vi "SenseQuiet_correct_final one.vi"() -> ()   [LabVIEW 2020]
uses:
  <vilib>/Platform/TimedLoop/XDataNode/timing_clust.ctl
  <vilib>/Platform/TimedLoop/XDataNode/nitl_modes.ctl
  <vilib>/Platform/TimedLoop/XDataNode/wakeup.ctl
  <vilib>/Instr/_visa.llb/VISA Configure Serial Port (Instr).vi
  <vilib>/platform/TimedLoop/XDataNode/XDataNode.xnode
  <vilib>/Platform/TimedLoop/XDataNode/XDNodeRunTimeDep.lvlib
  <vilib>/ptbypt/NI_PtbyPt.lvlib
panel:
  in  "OLED Display Output":refnum<visa-resource-name>
  out "WARNING":string="Warning - Please be mindful of noise"
  out "VIOLATION":string="Violation! - Noise Level too high"
  out "WARNING":string="Warning - A Noise Persisting"
  out "CALIBRATING":string="Calibrating"
  out "Sound Waveform":dynamicdata(graph) caption="Sound Sensor Output"
  out "PIR Sensor":bool
  out "Light Sensor":bool
  in  "Case Structure Loop Stop":bool
  in  "Main Loop Stop":bool
  out "Violation Noise Elapsed Time":dbl caption="Elapsed Time (s)"
  out "Violation Threshold":dbl
  out "Warning Threshold":dbl
  out "Noise Floor":dbl
  out "Noise Level Over Time":dbl(graph)
  out "System Message":string
  out "Buzzer Active":bool
  out "Violation LED":bool
  out "Warning LED":bool
  out "Quiet LED":bool
  # "SenseQuiet"
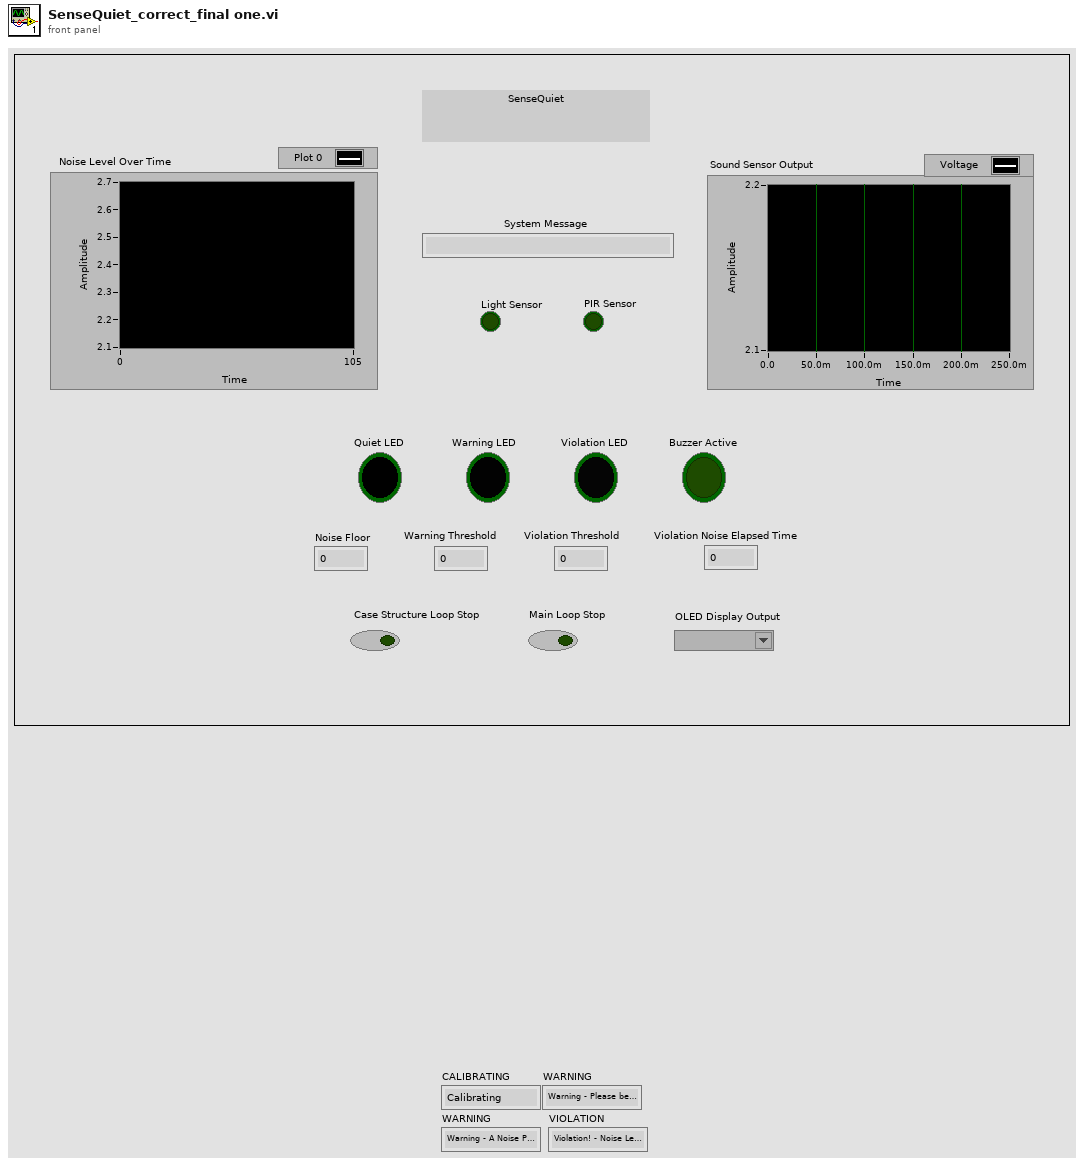
[diagram p1: front panel]
types:
  T1 = typedef "XDNodeRunTimeDep.lvlib/timing_clust.ctl" = cluster{"Expected End [f-1]":u64, "Actual End [f-1]":u64, "Finished Late? [f-1]":bool, "Expected End [i-1]":u64, "Actual End [i-1]":u64, "Finished Late? [i-1]":bool, "Expected Start [i]":u64, "Actual Start [i]":u64, "Expected Start [f]":u64, "Actual Start [f]":u64, "Source Name":string, "Structure Name":string, "Period":i64, "Deadline":i64, "Offset":i64, "Start":i64, "Priority":i32, "Timeout":i32, "Mode":T2, "Wakeup Reason":T3, "Error":errorcluster, "Source Type":string, "Secondary Source Type":string, "Global End Time":u64, "Global Start Time":u64, "Frame Duration":u64, "Iteration Duration":u64, "Assigned CPU":i32, "I/O Scan Engine Mode":u32}
  T2 = typedef "XDNodeRunTimeDep.lvlib/nitl_modes.ctl" = enum32{"No Change", "Process missed periods, maintain original phase", "Discard missed periods, maintain original phase", "Process missed periods, ignore original phase", "Discard missed periods, ignore original phase"}
  T3 = typedef "XDNodeRunTimeDep.lvlib/wakeup.ctl" = enum32{"Normal", "Aborted", "Asynchronous wakeup", "Timing source error", "Timed loop error", "Timeout"}
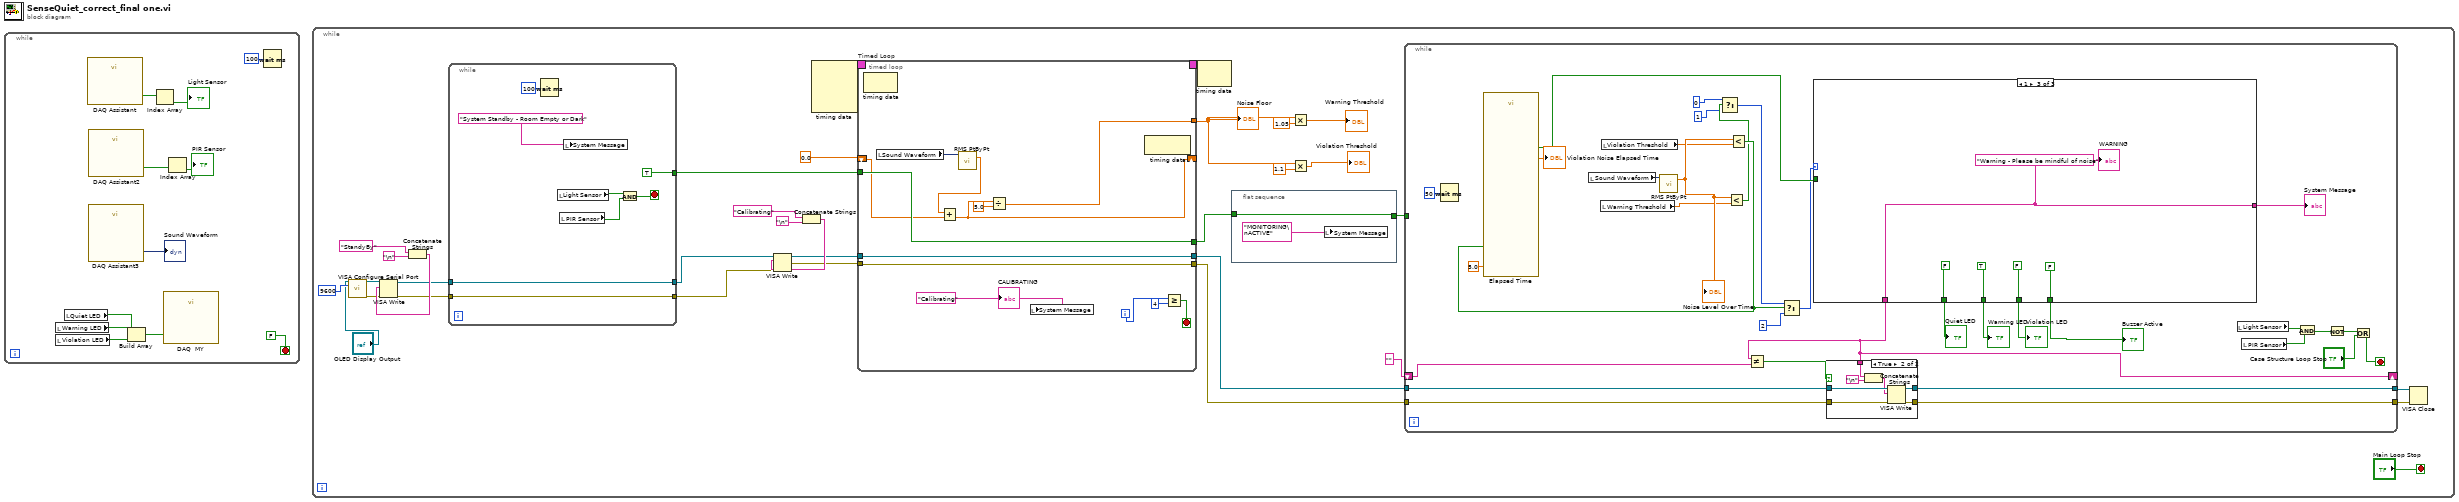
[diagram p0: block diagram]
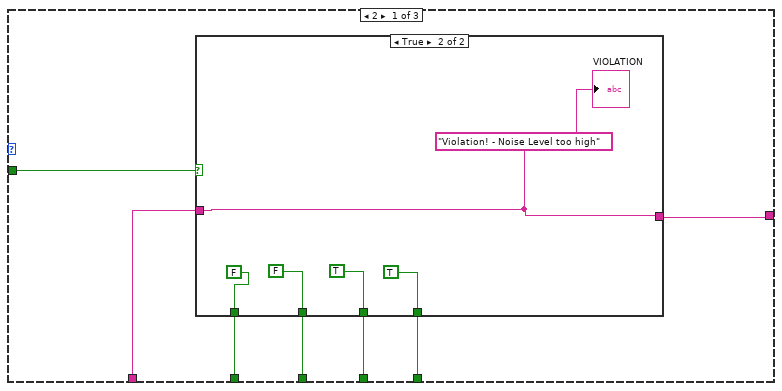
[diagram p3: hidden frame]
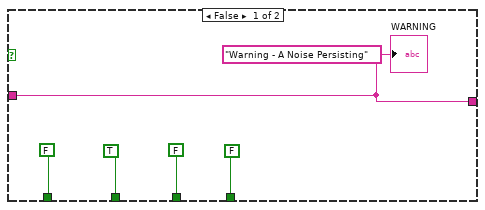
[diagram p4: hidden frame]
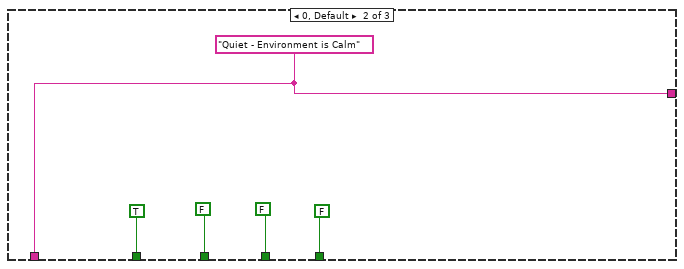
[diagram p5: hidden frame]
diagram:
  n1 = while {
    stop <- FALSE stop-if-true
    n2 = local read "Warning LED"() -> (w2:bool)
    n3 = local read "Violation LED"() -> (w1:bool)
    n4 = local read "Quiet LED"() -> (w4:bool)
    n5 = call "DAQ Assistant"() -> ("data"=w10:bool[])  [unwired: 17 in, 2 out]
    n6 = call "DAQ Assistant3"() -> ("data"=→"Sound Waveform":dynamicdata)  [unwired: 16 in, 3 out]
    n7 = call "DAQ Assistant2"() -> ("data"=w7:bool[])  [unwired: 17 in, 2 out]
    n8 = Build Array "Build Array"(w4, w2, w1) -> (w3:bool[])
    n9 = Index Array(array=w10) -> (element=→"Light Sensor":bool)  [unwired: 1 in]
    n10 = call "DAQ  MY"("data"=w3) -> ()  [unwired: 17 in, 2 out]
    n11 = Index Array(array=w7) -> (element=→"PIR Sensor":bool)  [unwired: 1 in]
    n12 = Wait (ms)(milliseconds to wait=u32 100) -> ()  [unwired: 1 out]
  }
  n13 = while {
    stop <- "Main Loop Stop" stop-if-true
    n14 = call-poly "VISA Configure Serial Port"("VISA resource name"="OLED Display Output", "baud rate (9600)"=u32 9600) -> ("VISA resource name out"=w25:refnum<visa-resource-name>, "error out"=w26:errorcluster)  [unwired: 12 in]
    n15 = Concatenate Strings("StandyBy", "\n") -> (w27:string)
    n16 = VISA Write(VISA resource name=w25, write buffer=w27, error in (no error)=w26) -> (VISA resource name out=w20:refnum<visa-resource-name>, error out=w21:errorcluster)  [unwired: 1 out]
    n17 = while {
      tunnel: [TRUE] -> w35
      tunnel: w21 -> [w45]
      tunnel: w20 -> [w46]
      tunnel: [w46] -> w18
      tunnel: [w45] -> w17
      stop <- w51 stop-if-true
      n18 = Wait (ms)(milliseconds to wait=u32 100) -> ()  [unwired: 1 out]
      n19 = local read "Light Sensor"() -> (w48:bool)
      n20 = local read "PIR Sensor"() -> (w50:bool)
      n21 = local write "System Message"("System Standby - Room Empty or Dark") -> ()
      n22 = And(x=w48, y=w50) -> (x .and. y?=w51:bool)
    }
    n23 = Concatenate Strings("Calibrating", "\n") -> (w31:string)
    n24 = VISA Write(VISA resource name=w18, write buffer=w31, error in (no error)=w17) -> (VISA resource name out=w28:refnum<visa-resource-name>, error out=w29:errorcluster)  [unwired: 1 out]
    n25 = node-c288() -> (w44:T1)  [unwired: 4 in]
    n26 = timed-loop "Timed Loop" {
      timing: w44 -> [_]
      timing-out: [_] -> w43
      tunnel: [w64] -> w39
      tunnel: w35 -> [w61]
      tunnel: [w61] -> w34
      shift-right: [w58] -> _
      shift-left: 0.0 -> [w59]
      tunnel: [w56] -> w15
      tunnel: w29 -> [w56]
      tunnel: [w55] -> w16
      tunnel: w28 -> [w55]
      i -> [w66]
      stop <- w63 stop-if-true
      w57 = "Calibrating"
      n27 = node-c288() -> ()  [unwired: 1 in, 1 out]
      n28 = local read "Sound Waveform"() -> (w60:dynamicdata)
      n29 = call <vilib>:"RMS PtByPt.vi"("x"=w60) -> ("rms value"=w62:dbl)  [unwired: 3 in, 1 out]
      n30 = Add(x=w62, y=w59) -> (x+y=w58:dbl)
      n31 = Divide(x=w58, y=5.0) -> (x/y=w64:dbl)
      n32 = local write "System Message"(w57) -> ()
      n33 = node-c288() -> ()  [unwired: 1 in, 1 out]
      n34 = Greater Or Equal?(x=w66, y=4) -> (x >= y?=w63:bool)
      "CALIBRATING" <- w57
    }
    "Noise Floor" <- w39
    n35 = node-c288(w43) -> ()  [unwired: 1 out]
    n36 = flat-sequence {
      tunnel: w34 -> [w53]
      tunnel: [w53] -> w37
      frame #0 {
        n37 = local write "System Message"("MONITORING\nACTIVE") -> ()
      }
    }
    n38 = Multiply(x=w39, y=1.05) -> (x*y=→"Warning Threshold":dbl)
    n39 = Multiply(x=w39, y=1.1) -> (x*y=→"Violation Threshold":dbl)
    n40 = while {
      tunnel: w37 -> [_]
      tunnel: w16 -> [w78]
      tunnel: w15 -> [w77]
      tunnel: [w76] -> w14
      tunnel: [w75] -> w13
      shift-right: [w74] -> _
      shift-left: "" -> [w73]
      stop <- w101 stop-if-true
      n41 = Wait (ms)(milliseconds to wait=u32 50) -> ()  [unwired: 1 out]
      n42 = local read "Sound Waveform"() -> (w81:dynamicdata)
      n43 = local read "Warning Threshold"() -> (w96:dbl)
      n44 = local read "Violation Threshold"() -> (w95:dbl)
      n45 = call <vilib>:"RMS PtByPt.vi"("x"=w81) -> ("rms value"=w100:dbl)  [unwired: 3 in, 1 out]
      "Noise Level Over Time" <- w100
      n46 = Less?(x=w100, y=w96) -> (x < y?=w92:bool)
      n47 = Select(t=0, s=w92, f=1) -> (s? t:f=w93:i32)
      n48 = Less?(x=w100, y=w95) -> (x < y?=w97:bool)
      n49 = call "Elapsed Time"("Time Target (s)"=5.0, "Reset"=w97) -> ("Elapsed Time (s)"=→"Violation Noise Elapsed Time":dbl, "Time has Elapsed"=w98:bool)  [unwired: 10 in, 6 out]
      n50 = Select(t=w93, s=w97, f=2) -> (s? t:f=w94:i32)
      n51 = case shown="1" w94 {
        tunnel: [w120 w131 w136] -> w85
        tunnel: w98 -> [w119 _ _]
        tunnel: [w118 TRUE FALSE] -> w80
        tunnel: [w117 FALSE TRUE] -> w87
        tunnel: [w116 FALSE FALSE] -> w86
        tunnel: [w115 FALSE FALSE] -> w79
        tunnel: [w114 w131 w136] -> w74
        frame 2 {
          n52 = case shown="True" w119 {
            tunnel: [w121 w126] -> w120
            tunnel: [FALSE FALSE] -> w118
            tunnel: [TRUE FALSE] -> w117
            tunnel: [FALSE TRUE] -> w116
            tunnel: [FALSE TRUE] -> w115
            tunnel: [w121 w126] -> w114
            frame False {
              w121 = "Warning - A Noise Persisting"
              "WARNING" <- w121
            }
            frame True {
              w126 = "Violation! - Noise Level too high"
              "VIOLATION" <- w126
            }
          }
        }
        frame 0, Default {
          w131 = "Quiet - Environment is Calm"
        }
        frame 1 {
          w136 = "Warning - Please be mindful of noise"
          "WARNING" <- w136
        }
      }
      "Quiet LED" <- w80
      "Warning LED" <- w87
      "Violation LED" <- w86
      "Buzzer Active" <- w79
      "System Message" <- w85
      n53 = Not Equal?(x=w74, y=w73) -> (x != y?=w72:bool)
      n54 = case shown="True" w72 {
        tunnel: w78 -> [w106 w113]
        tunnel: w77 -> [w105 w112]
        tunnel: [w106 w109] -> w76
        tunnel: [w105 w108] -> w75
        tunnel: w74 -> [_ w107]
        frame False {
        }
        frame True {
          n55 = Concatenate Strings(w107, "\n") -> (w110:string)
          n56 = VISA Write(VISA resource name=w113, write buffer=w110, error in (no error)=w112) -> (VISA resource name out=w109:refnum<visa-resource-name>, error out=w108:errorcluster)  [unwired: 1 out]
        }
      }
      n57 = local read "Light Sensor"() -> (w82:bool)
      n58 = local read "PIR Sensor"() -> (w104:bool)
      n59 = And(x=w82, y=w104) -> (x .and. y?=w83:bool)
      n60 = Not(x=w83) -> (.not. x?=w84:bool)
      n61 = Or(x=w84, y="Case Structure Loop Stop") -> (x .or. y?=w101:bool)
    }
    n62 = VISA Close(VISA resource name=w14, error in (no error)=w13) -> ()  [unwired: 1 out]
  }
